vi "Run Bfr Tx - FIFO Count Packets.vi"(8 "error in (no error)":errorcluster, 11 "Packet Count (t-1)":dbl) -> (0 "error out":errorcluster, 3 "Packet Count (t)":dbl)   [LabVIEW 2019, in "UDP-Custom-Device Engine.lvlib"]
uses:
  UDP-Custom-Device Engine.lvlib
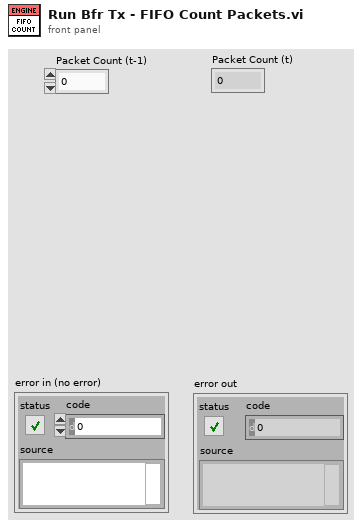
[diagram p1: front panel]
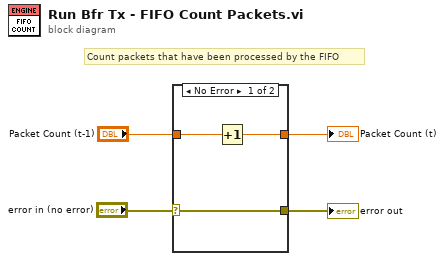
[diagram p0: block diagram]
diagram:
  # "Count packets that have been processed by the FIFO"
  n1 = case shown="No Error" "error in (no error)" {
    selector: "error in (no error)" -> [w7 w9]
    tunnel: [w7 w9] -> w3
    tunnel: "Packet Count (t-1)" -> [w6 w8]
    tunnel: [w5 w8] -> w1
    frame No Error {
      n2 = Increment(x=w6) -> (x+1=w5:dbl)
    }
    frame Error {
    }
  }
  "error out" <- w3
  "Packet Count (t)" <- w1
